vi "readCNT.vi"(8 "error in (no error)":errorcluster, 11 "CNT90 in":refnum<class "CNT90.lvclass">) -> (0 "error out":errorcluster, 2 "medicion":dbl, 3 "CNT90 out":refnum<class "CNT90.lvclass">)   [LabVIEW 2019, in "CNT90.lvclass"]
uses:
  CNT90.lvclass
panel:
  out "read buffer":string
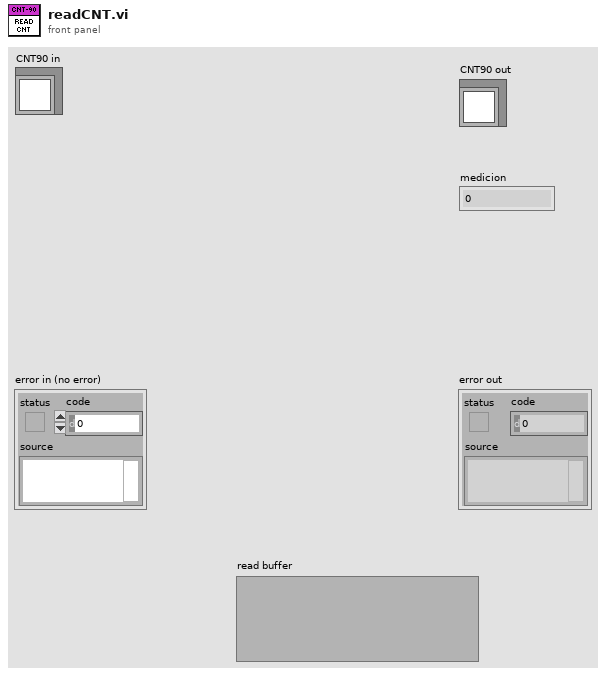
[diagram p1: front panel]
types:
  T1 = cluster{"error":bool, "code":i32, "source":string}
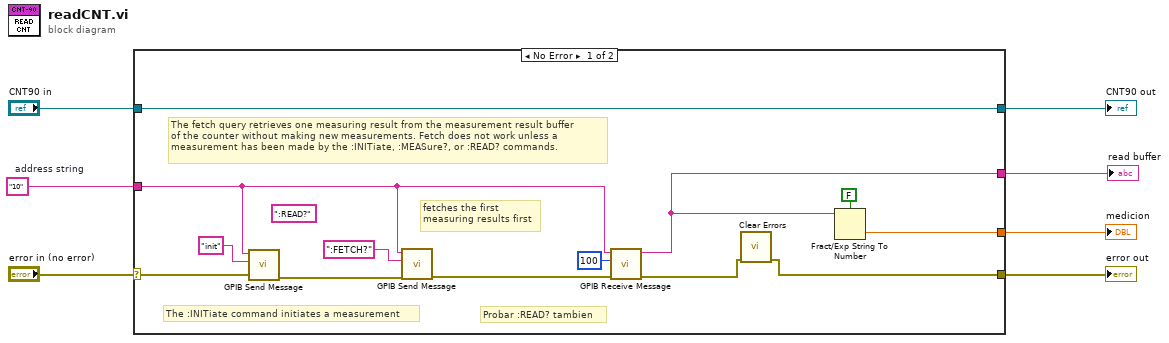
[diagram p0: block diagram]
diagram:
  w3 = "10"  # address string
  n1 = case shown="No Error" "error in (no error)" {
    selector: "error in (no error)" -> [w15 w22]
    tunnel: [w10 w22] -> w6
    tunnel: [w20 w21] -> w5
    tunnel: "CNT90 in" -> [w20 w21]
    tunnel: w3 -> [w14 _]
    tunnel: [w13 _] -> w2
    tunnel: [w12 _] -> w1
    frame No Error {
      (unwired) ":READ?" ("write buffer")
      # "Probar :READ? tambien"
      # "The :INITiate command initiates a measurement"
      # "The fetch query retrieves one measuring result from the measurement result buffer\nof the counter without making new measurements. Fetch does not work unless a\nmeasurement has been made by the :INITiate, :MEASure?, or :READ? commands."
      # "fetches the first\nmeasuring results first"
      n2 = call <instrlib>:"GPIB Send Message.vi"("address string"=w14, "write buffer"="init", "error in"=w15) -> ("error out"=w18:T1)  [unwired: 4 in, 2 out]
      n3 = call <instrlib>:"GPIB Send Message.vi"("address string"=w14, "write buffer"=":FETCH?", "error in"=w18) -> ("error out"=w16:T1)  [unwired: 4 in, 2 out]
      n4 = call <instrlib>:"GPIB Receive Message.vi"("address string"=w14, "byte count"=100, "error in"=w16) -> ("read buffer"=w12:string, "error out"=w11:T1)  [unwired: 4 in, 1 out]
      n5 = call <vilib>:"Clear Errors.vi"("error in (no error)"=w11) -> ("error out"=w10:errorcluster)  [unwired: 5 in, 1 out]
      n6 = Fract/Exp String To Number(use system decimal point (T)=FALSE, string=w12) -> (number=w13:dbl)  [unwired: 2 in, 1 out]
    }
    frame Error {
    }
  }
  "error out" <- w6
  "CNT90 out" <- w5
  "medicion" <- w2
  "read buffer" <- w1
